vi "CheezyAtan2.vi"(1 "arg2":dbl, 2 "arg1":dbl) -> (0 "atan2(arg1, arg2)":dbl)   [LabVIEW 2016]
uses:
  <userlib>/836-Libraries/Math/CheezyMath/MathConstantsNames.ctl
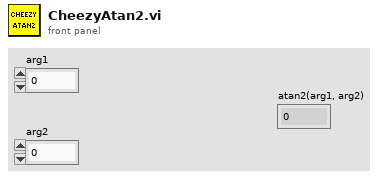
[diagram p1: front panel]
types:
  T1 = typedef "MathConstantsNames.ctl" = enum16{"sq2p1", "sq2m1", "p4", "p3", "p2", "p1", "p0", "q4", "q3", "q2", "q1", "q0", "PIO2"}
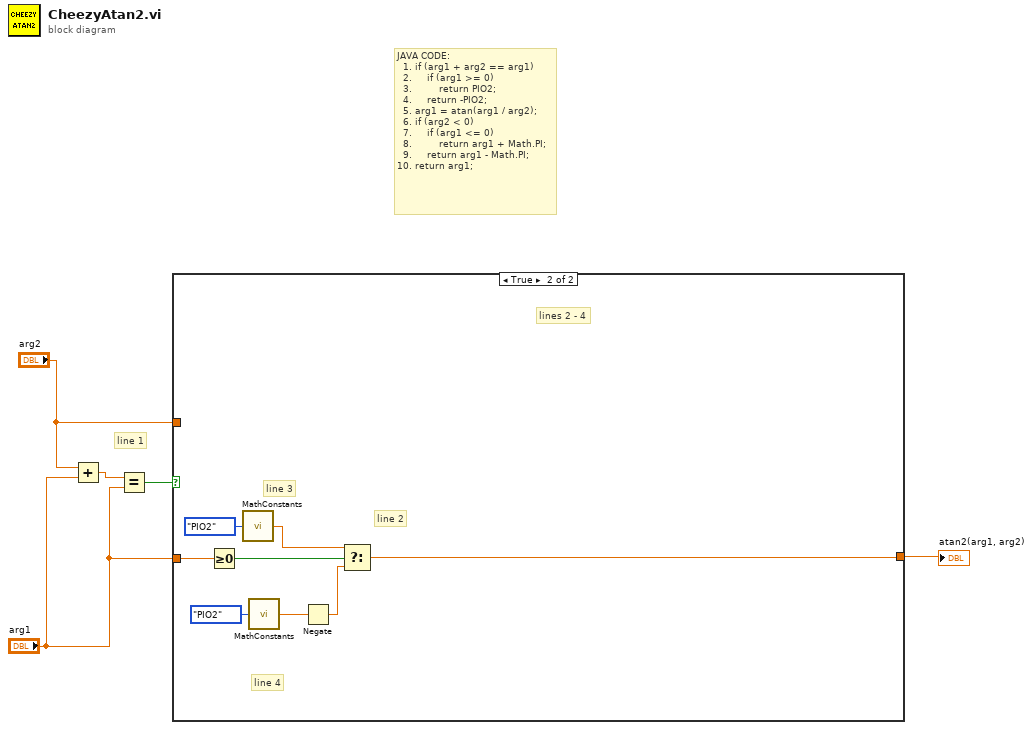
[diagram p0: block diagram]
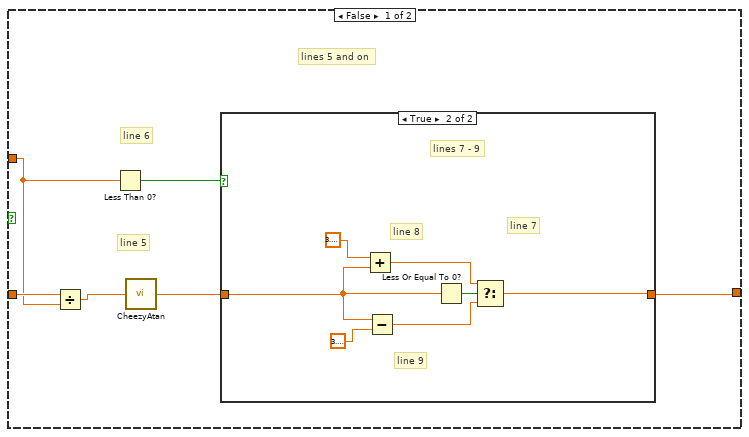
[diagram p2: hidden frame]
diagram:
  # "line 1"
  # "JAVA CODE:\n  1. if (arg1 + arg2 == arg1)\n  2.     if (arg1 >= 0)\n  3.         return PIO2;\n  4.     return -PIO2;\n  5. arg1 = atan(arg1 / arg2);\n  6. if (arg2 < 0)\n  7.     if (arg1 <= 0)\n  8.         return arg1 + Math.PI;\n  9.     return arg1 - Math.PI;\n10. return arg1;"
  n1 = Add(x="arg2", y="arg1") -> (x+y=w5:dbl)
  n2 = Equal?(x=w5, y="arg1") -> (x = y?=w4:bool)
  n3 = case shown="True" w4 {
    tunnel: "arg1" -> [w11 w27]
    tunnel: [w6 w20] -> w2
    tunnel: "arg2" -> [w9 _]
    frame False {
      # "line 6"
      # "line 5"
      # "lines 5 and on"
      n4 = Divide(x=w11, y=w9) -> (x/y=w10:dbl)
      n5 = Less Than 0?(x=w9) -> (x < 0?=w8:bool)
      n6 = call <userlib>:"CheezyAtan.vi"("arg"=w10) -> ("atan(arg)"=w7:dbl)
      n7 = case shown="True" w8 {
        tunnel: w7 -> [w12 w16]
        tunnel: [w12 w13] -> w6
        frame False {
          # "line 10"
        }
        frame True {
          # "line 8"
          # "line 9"
          # "line 7"
          # "lines 7 - 9"
          n8 = Add(x=3.141592653589793, y=w16) -> (x+y=w17:dbl)
          n9 = Subtract(x=w16, y=3.141592653589793) -> (x-y=w14:dbl)
          n10 = Less Or Equal To 0?(x=w16) -> (x <= 0?=w19:bool)
          n11 = Select(t=w17, s=w19, f=w14) -> (s? t:f=w13:dbl)
        }
      }
    }
    frame True {
      # "line 4"
      # "line 3"
      # "line 2"
      # "lines 2 - 4"
      n12 = Greater Or Equal To 0?(x=w27) -> (x >= 0?=w26:bool)
      n13 = call <userlib>:"MathConstants.vi"("Constant Name"=MathConstantsNames."PIO2") -> ("Constant Value"=w25:dbl)
      n14 = call <userlib>:"MathConstants.vi"("Constant Name"=MathConstantsNames."PIO2") -> ("Constant Value"=w22:dbl)
      n15 = Negate(x=w22) -> (-x=w21:dbl)
      n16 = Select(t=w25, s=w26, f=w21) -> (s? t:f=w20:dbl)
    }
  }
  "atan2(arg1, arg2)" <- w2
